vi "Loop_Timing_Slow_Loop.vi"(8 "error in":errorcluster, 11 "Controller Select":T1(ring)=enum."100hz/100hz" caption="Enum") -> (0 "error out":errorcluster, 2 "Iteration Count":dbl, 3 "Change Control Counter":dbl, 4 "Hz":dbl format="%#_4g")   [LabVIEW 2014]
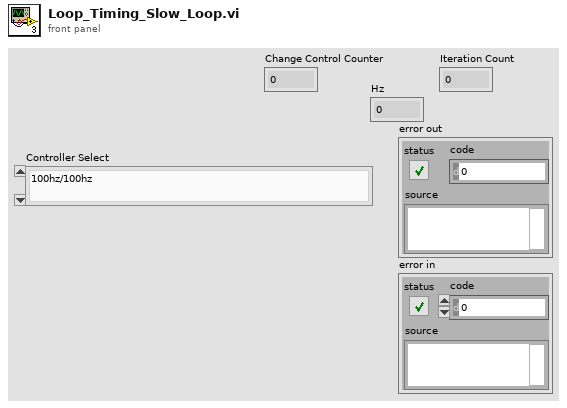
[diagram p1: front panel]
types:
  T1 = enum16{"100hz/50hz", "100hz/100hz", "200hz/200hz", "200hz/20hz", "User Defined"}
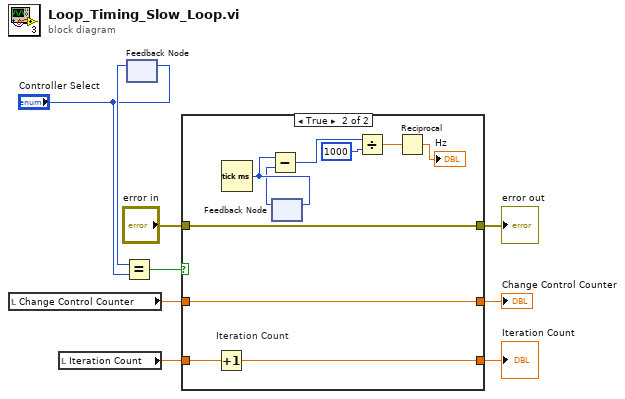
[diagram p0: block diagram]
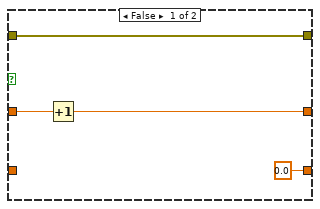
[diagram p2: hidden frame]
diagram:
  n1 = local read "Change Control Counter"() -> (w4:dbl)
  n2 = local read "Iteration Count"() -> (w2:dbl)
  n3 = feedback #1() -> (w6:T1)  [unwired: 1 in]
  n4 = Equal?(x=w6, y="Controller Select") -> (x = y?=w7:bool)
  n5 = feedback-in #1("Controller Select") -> ()
  n6 = case shown="True" w7 {
    tunnel: "error in" -> [w13 w14]
    tunnel: [w13 w14] -> w8
    tunnel: [w12 w23] -> w5
    tunnel: w4 -> [w11 w23]
    tunnel: [0.0 ("Iteration Count") w22] -> w3
    tunnel: w2 -> [_ w21]
    frame False {
      n7 = Increment(x=w11) -> (x+1=w12:dbl)
    }
    frame True {
      n8 = Increment "Iteration Count"(x=w21) -> (x+1=w22:dbl)
      n9 = Tick Count (ms)() -> (millisecond timer value=w20:u32)
      n10 = feedback-in #2(w20) -> ()
      n11 = feedback #2() -> (w19:u32)  [unwired: 1 in]
      n12 = Subtract(x=w20, y=w19) -> (x-y=w18:u32)
      n13 = Divide(x=w18, y=u32 1000) -> (x/y=w16:dbl)
      n14 = Reciprocal(x=w16) -> (1/x=→"Hz":dbl)
    }
  }
  "error out" <- w8
  "Change Control Counter" <- w5
  "Iteration Count" <- w3
